vi "HandleObservationSync.vi"(8 "error in (no error)":errorcluster, 11 "S4GUI in":refnum<class "S4GUI.lvclass">) -> (0 "error out":errorcluster, 3 "S4GUI out":refnum<class "S4GUI.lvclass">)   [LabVIEW 2018, in "S4GUI.lvclass"] (continued)
          n1824 = call-dynamic "Read enabled.vi"("error in (no error)"=w5050, "Server in"=w5052) -> ("error out"=w5049:errorcluster, "enabled"=w5048:bool, "Server out"=w5051:refnum<class "Acquisition.lvclass">)  [unwired: 7 in]
          n1825 = case shown="True" w5048 {
            tunnel: [w5106 w5114] -> w5073
            tunnel: [w5107 w5113] -> w5071
            tunnel: w5051 -> [w5107 w5111]
            tunnel: w5049 -> [w5106 w5110]
            frame False {
            }
            frame True {
              n1826 = call-dynamic "Read Channel.vi"("error in (no error)"=w5110, "Acquisition in"=w5111) -> ("error out"=w5118:errorcluster, "Channel.lvclass"=w5119:refnum<class "Channel.lvclass">, "Acquisition out"=w5112:refnum<class "Acquisition.lvclass">)  [unwired: 7 in]
              n1827 = call-dynamic "Read State Machine.vi"("error in (no error)"=w5118, "Device in"=w5119) -> ("error out"=w5117:errorcluster, "State Machine.lvclass"=w5115:refnum<class "State Machine.lvclass">, "Device out"=w5121:refnum<class "Channel.lvclass">)  [unwired: 7 in]
              n1828 = call "Next State.vi"("error in (no error)"=w5117, "New_State"=58, "State Machine in"=w5115) -> ("error out"=w5109:errorcluster, "State Machine out"=w5108:refnum<class "State Machine.lvclass">)  [unwired: 7 in]
              n1829 = call-dynamic "Write State Machine.vi"("error in (no error)"=w5109, "State Machine.lvclass"=w5108, "Device in"=w5121) -> ("error out"=w5122:errorcluster, "Device out"=w5120:refnum<class "Channel.lvclass">)  [unwired: 7 in]
              n1830 = call-dynamic "Write Channel.vi"("error in (no error)"=w5122, "Channel.lvclass"=w5120, "Acquisition in"=w5112) -> ("error out"=w5114:errorcluster, "Acquisition out"=w5113:refnum<class "Acquisition.lvclass">)  [unwired: 7 in]
            }
          }
          n1831 = call-dynamic "Write AcquisitionC.vi"("error in (no error)"=w5073, "Acquisition.lvclass"=w5071, "S4ACS_GUI in"=w5072) -> ("error out"=w5067:errorcluster, "S4ACS_GUI out"=w5066:refnum<class "S4GUI.lvclass">)  [unwired: 7 in]
          n1832 = call-dynamic "Read AcquisitionD.vi"("error in (no error)"=w5067, "S4ACS_GUI in"=w5066) -> ("error out"=w5045:errorcluster, "Acquisition.lvclass"=w5047:refnum<class "Acquisition.lvclass">, "S4ACS_GUI out"=w5065:refnum<class "S4GUI.lvclass">)  [unwired: 7 in]
          n1833 = call-dynamic "Read enabled.vi"("error in (no error)"=w5045, "Server in"=w5047) -> ("error out"=w5044:errorcluster, "enabled"=w5043:bool, "Server out"=w5046:refnum<class "Acquisition.lvclass">)  [unwired: 7 in]
          n1834 = case shown="True" w5043 {
            tunnel: w5044 -> [w5089 w5105]
            tunnel: [w5089 w5104] -> w5068
            tunnel: w5046 -> [w5090 w5095]
            tunnel: [w5090 w5093] -> w5064
            frame False {
            }
            frame True {
              n1835 = call-dynamic "Read Channel.vi"("error in (no error)"=w5105, "Acquisition in"=w5095) -> ("error out"=w5100:errorcluster, "Channel.lvclass"=w5099:refnum<class "Channel.lvclass">, "Acquisition out"=w5094:refnum<class "Acquisition.lvclass">)  [unwired: 7 in]
              n1836 = call-dynamic "Read State Machine.vi"("error in (no error)"=w5100, "Device in"=w5099) -> ("error out"=w5101:errorcluster, "State Machine.lvclass"=w5103:refnum<class "State Machine.lvclass">, "Device out"=w5097:refnum<class "Channel.lvclass">)  [unwired: 7 in]
              n1837 = call "Next State.vi"("error in (no error)"=w5101, "New_State"=58, "State Machine in"=w5103) -> ("error out"=w5091:errorcluster, "State Machine out"=w5092:refnum<class "State Machine.lvclass">)  [unwired: 7 in]
              n1838 = call-dynamic "Write State Machine.vi"("error in (no error)"=w5091, "State Machine.lvclass"=w5092, "Device in"=w5097) -> ("error out"=w5096:errorcluster, "Device out"=w5098:refnum<class "Channel.lvclass">)  [unwired: 7 in]
              n1839 = call-dynamic "Write Channel.vi"("error in (no error)"=w5096, "Channel.lvclass"=w5098, "Acquisition in"=w5094) -> ("error out"=w5104:errorcluster, "Acquisition out"=w5093:refnum<class "Acquisition.lvclass">)  [unwired: 7 in]
            }
          }
          n1840 = call-dynamic "Write AcquisitionD.vi"("error in (no error)"=w5068, "Acquisition.lvclass"=w5064, "S4ACS_GUI in"=w5065) -> ("error out"=w5042:errorcluster, "S4ACS_GUI out"=w5063:refnum<class "S4GUI.lvclass">)  [unwired: 7 in]
          n1841 = flat-sequence {
            tunnel: w5042 -> [w5087]
            tunnel: [w5087] -> w5041
            frame #0 {
              n1842 = Tick Count (ms)() -> (millisecond timer value=→"time9":u32)
            }
          }
          n1843 = Increment(x=w5081) -> (x+1=w5080:u32)
          n1844 = Bundle By Name(cluster=w5063, "Obs_state"=w5080) -> (w5079:refnum<class "S4GUI.lvclass">)
        }
        frame 363 {
          # "T: mode EXPOSE\nF: mode FIRE\nNa seq de foco, só \ndeve usar mode EXPOSE."
          # "Espera todos os canais chegarem ao estado de repouso.\n(estado 0  de Channel:Run.vi)."
          n1845 = call-dynamic "Read AcquisitionA.vi"("error in (no error)"=w5207, "S4ACS_GUI in"=w5208) -> ("error out"=w5186:errorcluster, "Acquisition.lvclass"=w5187:refnum<class "Acquisition.lvclass">, "S4ACS_GUI out"=w5210:refnum<class "S4GUI.lvclass">)  [unwired: 7 in]
          n1846 = call-dynamic "Read enabled.vi"("error in (no error)"=w5186, "Server in"=w5187) -> ("error out"=w5188:errorcluster, "enabled"=w5190:bool, "Server out"=w5189:refnum<class "Acquisition.lvclass">)  [unwired: 7 in]
          n1847 = case shown="True" w5190 {
            tunnel: [w5284 w5302] -> w5211
            tunnel: [w5283 w5301] -> w5209
            tunnel: w5189 -> [w5284 w5294]
            tunnel: w5188 -> [w5283 w5293]
            tunnel: [TRUE w5286] -> w5167
            tunnel: [FALSE w5287] -> w5163
            frame False {
            }
            frame True {
              n1848 = call-dynamic "Read Channel.vi"("error in (no error)"=w5293, "Acquisition in"=w5294) -> ("error out"=w5290:errorcluster, "Channel.lvclass"=w5291:refnum<class "Channel.lvclass">, "Acquisition out"=w5303:refnum<class "Acquisition.lvclass">)  [unwired: 7 in]
              n1849 = call-dynamic "Read wait_expose.vi"("error in (no error)"=w5290, "Channel in"=w5291) -> ("error out"=w5288:errorcluster, "wait_expose"=w5287:bool, "Channel out"=w5289:refnum<class "Channel.lvclass">)  [unwired: 7 in]
              n1850 = call-dynamic "Read State Machine.vi"("error in (no error)"=w5288, "Device in"=w5289) -> ("error out"=w5295:errorcluster, "State Machine.lvclass"=w5297:refnum<class "State Machine.lvclass">, "Device out"=w5299:refnum<class "Channel.lvclass">)  [unwired: 7 in]
              n1851 = call-dynamic "Read State.vi"("error in (no error)"=w5295, "State Machine in"=w5297) -> ("error out"=w5292:errorcluster, "State"=w5285:i32, "State Machine out"=w5296:refnum<class "State Machine.lvclass">)  [unwired: 7 in]
              n1852 = Equal To 0?(x=w5285) -> (x = 0?=w5286:bool)
              n1853 = call-dynamic "Write State Machine.vi"("error in (no error)"=w5292, "State Machine.lvclass"=w5296, "Device in"=w5299) -> ("error out"=w5298:errorcluster, "Device out"=w5300:refnum<class "Channel.lvclass">)  [unwired: 7 in]
              n1854 = call-dynamic "Write Channel.vi"("error in (no error)"=w5298, "Channel.lvclass"=w5300, "Acquisition in"=w5303) -> ("error out"=w5301:errorcluster, "Acquisition out"=w5302:refnum<class "Acquisition.lvclass">)  [unwired: 7 in]
            }
          }
          n1855 = call-dynamic "Write AcquisitionA.vi"("error in (no error)"=w5209, "Acquisition.lvclass"=w5211, "S4ACS_GUI in"=w5210) -> ("error out"=w5203:errorcluster, "S4ACS_GUI out"=w5204:refnum<class "S4GUI.lvclass">)  [unwired: 7 in]
          n1856 = call "Read AcquisitionB.vi"("error in (no error)"=w5203, "S4ACS_GUI in"=w5204) -> ("error out"=w5183:errorcluster, "Acquisition.lvclass"=w5185:refnum<class "Acquisition.lvclass">, "S4ACS_GUI out"=w5201:refnum<class "S4GUI.lvclass">)  [unwired: 7 in]
          n1857 = call-dynamic "Read enabled.vi"("error in (no error)"=w5183, "Server in"=w5185) -> ("error out"=w5182:errorcluster, "enabled"=w5181:bool, "Server out"=w5184:refnum<class "Acquisition.lvclass">)  [unwired: 7 in]
          n1858 = case shown="True" w5181 {
            tunnel: w5184 -> [w5261 w5280]
            tunnel: w5182 -> [w5260 w5279]
            tunnel: [w5261 w5277] -> w5202
            tunnel: [w5260 w5276] -> w5200
            tunnel: [TRUE w5268] -> w5166
            tunnel: [FALSE ("expose") w5262] -> w5162
            frame False {
            }
            frame True {
              n1859 = call-dynamic "Read Channel.vi"("error in (no error)"=w5279, "Acquisition in"=w5280) -> ("error out"=w5264:errorcluster, "Channel.lvclass"=w5266:refnum<class "Channel.lvclass">, "Acquisition out"=w5278:refnum<class "Acquisition.lvclass">)  [unwired: 7 in]
              n1860 = call-dynamic "Read wait_expose.vi"("error in (no error)"=w5264, "Channel in"=w5266) -> ("error out"=w5263:errorcluster, "wait_expose"=w5262:bool, "Channel out"=w5265:refnum<class "Channel.lvclass">)  [unwired: 7 in]
              n1861 = call-dynamic "Read State Machine.vi"("error in (no error)"=w5263, "Device in"=w5265) -> ("error out"=w5270:errorcluster, "State Machine.lvclass"=w5272:refnum<class "State Machine.lvclass">, "Device out"=w5274:refnum<class "Channel.lvclass">)  [unwired: 7 in]
              n1862 = call-dynamic "Read State.vi"("error in (no error)"=w5270, "State Machine in"=w5272) -> ("error out"=w5269:errorcluster, "State"=w5267:i32, "State Machine out"=w5271:refnum<class "State Machine.lvclass">)  [unwired: 7 in]
              n1863 = Equal To 0?(x=w5267) -> (x = 0?=w5268:bool)
              n1864 = call-dynamic "Write State Machine.vi"("error in (no error)"=w5269, "State Machine.lvclass"=w5271, "Device in"=w5274) -> ("error out"=w5273:errorcluster, "Device out"=w5275:refnum<class "Channel.lvclass">)  [unwired: 7 in]
              n1865 = call-dynamic "Write Channel.vi"("error in (no error)"=w5273, "Channel.lvclass"=w5275, "Acquisition in"=w5278) -> ("error out"=w5276:errorcluster, "Acquisition out"=w5277:refnum<class "Acquisition.lvclass">)  [unwired: 7 in]
            }
          }
          n1866 = call "Write AcquisitionB.vi"("error in (no error)"=w5200, "Acquisition.lvclass"=w5202, "S4ACS_GUI in"=w5201) -> ("error out"=w5196:errorcluster, "S4ACS_GUI out"=w5195:refnum<class "S4GUI.lvclass">)  [unwired: 7 in]
          n1867 = call-dynamic "Read AcquisitionC.vi"("error in (no error)"=w5196, "S4ACS_GUI in"=w5195) -> ("error out"=w5178:errorcluster, "Acquisition.lvclass"=w5180:refnum<class "Acquisition.lvclass">, "S4ACS_GUI out"=w5198:refnum<class "S4GUI.lvclass">)  [unwired: 7 in]
          n1868 = call-dynamic "Read enabled.vi"("error in (no error)"=w5178, "Server in"=w5180) -> ("error out"=w5177:errorcluster, "enabled"=w5176:bool, "Server out"=w5179:refnum<class "Acquisition.lvclass">)  [unwired: 7 in]
          n1869 = case shown="True" w5176 {
            tunnel: [w5237 w5252] -> w5199
            tunnel: [w5238 w5251] -> w5197
            tunnel: w5179 -> [w5238 w5247]
            tunnel: w5177 -> [w5237 w5246]
            tunnel: [TRUE w5244] -> w5165
            tunnel: [FALSE ("expose") w5239] -> w5161
            frame False {
            }
            frame True {
              n1870 = call-dynamic "Read Channel.vi"("error in (no error)"=w5246, "Acquisition in"=w5247) -> ("error out"=w5241:errorcluster, "Channel.lvclass"=w5243:refnum<class "Channel.lvclass">, "Acquisition out"=w5250:refnum<class "Acquisition.lvclass">)  [unwired: 7 in]
              n1871 = call-dynamic "Read wait_expose.vi"("error in (no error)"=w5241, "Channel in"=w5243) -> ("error out"=w5240:errorcluster, "wait_expose"=w5239:bool, "Channel out"=w5242:refnum<class "Channel.lvclass">)  [unwired: 7 in]
              n1872 = call-dynamic "Read State Machine.vi"("error in (no error)"=w5240, "Device in"=w5242) -> ("error out"=w5248:errorcluster, "State Machine.lvclass"=w5256:refnum<class "State Machine.lvclass">, "Device out"=w5254:refnum<class "Channel.lvclass">)  [unwired: 7 in]
              n1873 = call-dynamic "Read State.vi"("error in (no error)"=w5248, "State Machine in"=w5256) -> ("error out"=w5249:errorcluster, "State"=w5245:i32, "State Machine out"=w5257:refnum<class "State Machine.lvclass">)  [unwired: 7 in]
              n1874 = Equal To 0?(x=w5245) -> (x = 0?=w5244:bool)
              n1875 = call-dynamic "Write State Machine.vi"("error in (no error)"=w5249, "State Machine.lvclass"=w5257, "Device in"=w5254) -> ("error out"=w5255:errorcluster, "Device out"=w5253:refnum<class "Channel.lvclass">)  [unwired: 7 in]
              n1876 = call-dynamic "Write Channel.vi"("error in (no error)"=w5255, "Channel.lvclass"=w5253, "Acquisition in"=w5250) -> ("error out"=w5252:errorcluster, "Acquisition out"=w5251:refnum<class "Acquisition.lvclass">)  [unwired: 7 in]
            }
          }
          n1877 = call-dynamic "Write AcquisitionC.vi"("error in (no error)"=w5199, "Acquisition.lvclass"=w5197, "S4ACS_GUI in"=w5198) -> ("error out"=w5175:errorcluster, "S4ACS_GUI out"=w5191:refnum<class "S4GUI.lvclass">)  [unwired: 7 in]
          n1878 = call-dynamic "Read AcquisitionD.vi"("error in (no error)"=w5175, "S4ACS_GUI in"=w5191) -> ("error out"=w5171:errorcluster, "Acquisition.lvclass"=w5174:refnum<class "Acquisition.lvclass">, "S4ACS_GUI out"=w5193:refnum<class "S4GUI.lvclass">)  [unwired: 7 in]
          n1879 = call-dynamic "Read enabled.vi"("error in (no error)"=w5171, "Server in"=w5174) -> ("error out"=w5172:errorcluster, "enabled"=w5170:bool, "Server out"=w5173:refnum<class "Acquisition.lvclass">)  [unwired: 7 in]
          n1880 = case shown="True" w5170 {
            tunnel: [w5215 w5233] -> w5194
            tunnel: [w5214 w5232] -> w5192
            tunnel: [TRUE w5222] -> w5164
            tunnel: w5173 -> [w5215 w5224]
            tunnel: w5172 -> [w5214 w5223]
            tunnel: [FALSE ("expose") w5216] -> w5160
            frame False {
            }
            frame True {
              n1881 = call-dynamic "Read Channel.vi"("error in (no error)"=w5223, "Acquisition in"=w5224) -> ("error out"=w5218:errorcluster, "Channel.lvclass"=w5220:refnum<class "Channel.lvclass">, "Acquisition out"=w5234:refnum<class "Acquisition.lvclass">)  [unwired: 7 in]
              n1882 = call-dynamic "Read wait_expose.vi"("error in (no error)"=w5218, "Channel in"=w5220) -> ("error out"=w5217:errorcluster, "wait_expose"=w5216:bool, "Channel out"=w5219:refnum<class "Channel.lvclass">)  [unwired: 7 in]
              n1883 = call-dynamic "Read State Machine.vi"("error in (no error)"=w5217, "Device in"=w5219) -> ("error out"=w5226:errorcluster, "State Machine.lvclass"=w5228:refnum<class "State Machine.lvclass">, "Device out"=w5230:refnum<class "Channel.lvclass">)  [unwired: 7 in]
              n1884 = call-dynamic "Read State.vi"("error in (no error)"=w5226, "State Machine in"=w5228) -> ("error out"=w5225:errorcluster, "State"=w5221:i32, "State Machine out"=w5227:refnum<class "State Machine.lvclass">)  [unwired: 7 in]
              n1885 = Equal To 0?(x=w5221) -> (x = 0?=w5222:bool)
              n1886 = call-dynamic "Write State Machine.vi"("error in (no error)"=w5225, "State Machine.lvclass"=w5227, "Device in"=w5230) -> ("error out"=w5229:errorcluster, "Device out"=w5231:refnum<class "Channel.lvclass">)  [unwired: 7 in]
              n1887 = call-dynamic "Write Channel.vi"("error in (no error)"=w5229, "Channel.lvclass"=w5231, "Acquisition in"=w5234) -> ("error out"=w5232:errorcluster, "Acquisition out"=w5233:refnum<class "Acquisition.lvclass">)  [unwired: 7 in]
            }
          }
          n1888 = call-dynamic "Write AcquisitionD.vi"("error in (no error)"=w5192, "Acquisition.lvclass"=w5194, "S4ACS_GUI in"=w5193) -> ("error out"=w5158:errorcluster, "S4ACS_GUI out"=w5159:refnum<class "S4GUI.lvclass">)  [unwired: 7 in]
          n1889 = Compound Arithmetic op=OR(w5163, w5162, w5161, w5160) -> ()  [unwired: 1 out]
          n1890 = Compound Arithmetic op=AND(w5167, w5166, w5165, w5164) -> (w5168:bool)
          n1891 = Increment(x=w5169) -> (x+1=w5157:u32)
          n1892 = Select(t=w5157, s=w5168, f=w5169) -> (s? t:f=w5205:u32)
          n1893 = Bundle By Name(cluster=w5159, "Obs_state"=w5205) -> (w5206:refnum<class "S4GUI.lvclass">)
        }
        frame 364 {
          n1894 = flat-sequence {
            tunnel: [w5317] -> w5305
            tunnel: w5306 -> [w5317]
            tunnel: [w5313] -> w5304
            frame #0 {
              # "Espera 2s desde que enviou o comando\nWRITE_HEADER_DATA para os ACS"
              n1895 = local read "time9"() -> (w5312:u32)
              n1896 = Tick Count (ms)() -> (millisecond timer value=w5316:u32)
              "time 10" <- w5316
              n1897 = Subtract(x=w5316, y=w5312) -> (x-y=w5315:u32)
              "delay 89" <- w5315
              n1898 = Greater?(x=w5315, y=u32 2000) -> (0:w5313:bool)
            }
          }
          n1899 = Increment(x=w5309) -> (x+1=w5308:u32)
          n1900 = Select(t=w5308, s=w5304, f=w5309) -> (s? t:f=w5310:u32)
          n1901 = Bundle By Name(cluster=w5307, "Obs_state"=w5310) -> (w5311:refnum<class "S4GUI.lvclass">)
        }
        frame 365 {
          n1902 = call-dynamic "Read AcquisitionA.vi"("error in (no error)"=w5358, "S4ACS_GUI in"=w5359) -> ("error out"=w5334:errorcluster, "Acquisition.lvclass"=w5337:refnum<class "Acquisition.lvclass">, "S4ACS_GUI out"=w5361:refnum<class "S4GUI.lvclass">)  [unwired: 7 in]
          n1903 = call-dynamic "Read enabled.vi"("error in (no error)"=w5334, "Server in"=w5337) -> ("error out"=w5333:errorcluster, "enabled"=w5335:bool, "Server out"=w5336:refnum<class "Acquisition.lvclass">)  [unwired: 7 in]
          n1904 = case shown="True" w5335 {
            tunnel: w5336 -> [w5415 w5430]
            tunnel: w5333 -> [w5414 w5429]
            tunnel: [w5415 w5427] -> w5362
            tunnel: [w5414 w5426] -> w5360
            frame False {
            }
            frame True {
              n1905 = call-dynamic "Read Channel.vi"("error in (no error)"=w5429, "Acquisition in"=w5430) -> ("error out"=w5422:errorcluster, "Channel.lvclass"=w5421:refnum<class "Channel.lvclass">, "Acquisition out"=w5428:refnum<class "Acquisition.lvclass">)  [unwired: 7 in]
              n1906 = call-dynamic "Read State Machine.vi"("error in (no error)"=w5422, "Device in"=w5421) -> ("error out"=w5423:errorcluster, "State Machine.lvclass"=w5425:refnum<class "State Machine.lvclass">, "Device out"=w5419:refnum<class "Channel.lvclass">)  [unwired: 7 in]
              n1907 = call "Next State.vi"("error in (no error)"=w5423, "New_State"=50, "State Machine in"=w5425) -> ("error out"=w5416:errorcluster, "State Machine out"=w5417:refnum<class "State Machine.lvclass">)  [unwired: 7 in]
              n1908 = call-dynamic "Write State Machine.vi"("error in (no error)"=w5416, "State Machine.lvclass"=w5417, "Device in"=w5419) -> ("error out"=w5418:errorcluster, "Device out"=w5420:refnum<class "Channel.lvclass">)  [unwired: 7 in]
              n1909 = call-dynamic "Write Channel.vi"("error in (no error)"=w5418, "Channel.lvclass"=w5420, "Acquisition in"=w5428) -> ("error out"=w5426:errorcluster, "Acquisition out"=w5427:refnum<class "Acquisition.lvclass">)  [unwired: 7 in]
            }
          }
          n1910 = call-dynamic "Write AcquisitionA.vi"("error in (no error)"=w5360, "Acquisition.lvclass"=w5362, "S4ACS_GUI in"=w5361) -> ("error out"=w5353:errorcluster, "S4ACS_GUI out"=w5354:refnum<class "S4GUI.lvclass">)  [unwired: 7 in]
          n1911 = call "Read AcquisitionB.vi"("error in (no error)"=w5353, "S4ACS_GUI in"=w5354) -> ("error out"=w5330:errorcluster, "Acquisition.lvclass"=w5332:refnum<class "Acquisition.lvclass">, "S4ACS_GUI out"=w5351:refnum<class "S4GUI.lvclass">)  [unwired: 7 in]
          n1912 = call-dynamic "Read enabled.vi"("error in (no error)"=w5330, "Server in"=w5332) -> ("error out"=w5329:errorcluster, "enabled"=w5328:bool, "Server out"=w5331:refnum<class "Acquisition.lvclass">)  [unwired: 7 in]
          n1913 = case shown="True" w5328 {
            tunnel: w5331 -> [w5398 w5413]
            tunnel: w5329 -> [w5397 w5412]
            tunnel: [w5398 w5410] -> w5352
            tunnel: [w5397 w5409] -> w5350
            frame False {
            }
            frame True {
              n1914 = call-dynamic "Read Channel.vi"("error in (no error)"=w5412, "Acquisition in"=w5413) -> ("error out"=w5405:errorcluster, "Channel.lvclass"=w5404:refnum<class "Channel.lvclass">, "Acquisition out"=w5411:refnum<class "Acquisition.lvclass">)  [unwired: 7 in]
              n1915 = call-dynamic "Read State Machine.vi"("error in (no error)"=w5405, "Device in"=w5404) -> ("error out"=w5406:errorcluster, "State Machine.lvclass"=w5408:refnum<class "State Machine.lvclass">, "Device out"=w5402:refnum<class "Channel.lvclass">)  [unwired: 7 in]
              n1916 = call "Next State.vi"("error in (no error)"=w5406, "New_State"=50, "State Machine in"=w5408) -> ("error out"=w5399:errorcluster, "State Machine out"=w5400:refnum<class "State Machine.lvclass">)  [unwired: 7 in]
              n1917 = call-dynamic "Write State Machine.vi"("error in (no error)"=w5399, "State Machine.lvclass"=w5400, "Device in"=w5402) -> ("error out"=w5401:errorcluster, "Device out"=w5403:refnum<class "Channel.lvclass">)  [unwired: 7 in]
              n1918 = call-dynamic "Write Channel.vi"("error in (no error)"=w5401, "Channel.lvclass"=w5403, "Acquisition in"=w5411) -> ("error out"=w5409:errorcluster, "Acquisition out"=w5410:refnum<class "Acquisition.lvclass">)  [unwired: 7 in]
            }
          }
          n1919 = call "Write AcquisitionB.vi"("error in (no error)"=w5350, "Acquisition.lvclass"=w5352, "S4ACS_GUI in"=w5351) -> ("error out"=w5346:errorcluster, "S4ACS_GUI out"=w5345:refnum<class "S4GUI.lvclass">)  [unwired: 7 in]
          n1920 = call-dynamic "Read AcquisitionC.vi"("error in (no error)"=w5346, "S4ACS_GUI in"=w5345) -> ("error out"=w5325:errorcluster, "Acquisition.lvclass"=w5327:refnum<class "Acquisition.lvclass">, "S4ACS_GUI out"=w5348:refnum<class "S4GUI.lvclass">)  [unwired: 7 in]
          n1921 = call-dynamic "Read enabled.vi"("error in (no error)"=w5325, "Server in"=w5327) -> ("error out"=w5324:errorcluster, "enabled"=w5323:bool, "Server out"=w5326:refnum<class "Acquisition.lvclass">)  [unwired: 7 in]
          n1922 = case shown="True" w5323 {
            tunnel: [w5380 w5388] -> w5349
            tunnel: [w5381 w5387] -> w5347
            tunnel: w5326 -> [w5381 w5385]
            tunnel: w5324 -> [w5380 w5384]
            frame False {
            }
            frame True {
              n1923 = call-dynamic "Read Channel.vi"("error in (no error)"=w5384, "Acquisition in"=w5385) -> ("error out"=w5392:errorcluster, "Channel.lvclass"=w5393:refnum<class "Channel.lvclass">, "Acquisition out"=w5386:refnum<class "Acquisition.lvclass">)  [unwired: 7 in]
              n1924 = call-dynamic "Read State Machine.vi"("error in (no error)"=w5392, "Device in"=w5393) -> ("error out"=w5391:errorcluster, "State Machine.lvclass"=w5389:refnum<class "State Machine.lvclass">, "Device out"=w5395:refnum<class "Channel.lvclass">)  [unwired: 7 in]
              n1925 = call "Next State.vi"("error in (no error)"=w5391, "New_State"=50, "State Machine in"=w5389) -> ("error out"=w5383:errorcluster, "State Machine out"=w5382:refnum<class "State Machine.lvclass">)  [unwired: 7 in]
              n1926 = call-dynamic "Write State Machine.vi"("error in (no error)"=w5383, "State Machine.lvclass"=w5382, "Device in"=w5395) -> ("error out"=w5396:errorcluster, "Device out"=w5394:refnum<class "Channel.lvclass">)  [unwired: 7 in]
              n1927 = call-dynamic "Write Channel.vi"("error in (no error)"=w5396, "Channel.lvclass"=w5394, "Acquisition in"=w5386) -> ("error out"=w5388:errorcluster, "Acquisition out"=w5387:refnum<class "Acquisition.lvclass">)  [unwired: 7 in]
            }
          }
          n1928 = call-dynamic "Write AcquisitionC.vi"("error in (no error)"=w5349, "Acquisition.lvclass"=w5347, "S4ACS_GUI in"=w5348) -> ("error out"=w5343:errorcluster, "S4ACS_GUI out"=w5342:refnum<class "S4GUI.lvclass">)  [unwired: 7 in]
          n1929 = call-dynamic "Read AcquisitionD.vi"("error in (no error)"=w5343, "S4ACS_GUI in"=w5342) -> ("error out"=w5320:errorcluster, "Acquisition.lvclass"=w5322:refnum<class "Acquisition.lvclass">, "S4ACS_GUI out"=w5341:refnum<class "S4GUI.lvclass">)  [unwired: 7 in]
          n1930 = call-dynamic "Read enabled.vi"("error in (no error)"=w5320, "Server in"=w5322) -> ("error out"=w5319:errorcluster, "enabled"=w5318:bool, "Server out"=w5321:refnum<class "Acquisition.lvclass">)  [unwired: 7 in]
          n1931 = case shown="True" w5318 {
            tunnel: w5319 -> [w5363 w5379]
            tunnel: [w5363 w5378] -> w5344
            tunnel: w5321 -> [w5364 w5369]
            tunnel: [w5364 w5367] -> w5340
            frame False {
            }
            frame True {
              n1932 = call-dynamic "Read Channel.vi"("error in (no error)"=w5379, "Acquisition in"=w5369) -> ("error out"=w5374:errorcluster, "Channel.lvclass"=w5373:refnum<class "Channel.lvclass">, "Acquisition out"=w5368:refnum<class "Acquisition.lvclass">)  [unwired: 7 in]
              n1933 = call-dynamic "Read State Machine.vi"("error in (no error)"=w5374, "Device in"=w5373) -> ("error out"=w5375:errorcluster, "State Machine.lvclass"=w5377:refnum<class "State Machine.lvclass">, "Device out"=w5371:refnum<class "Channel.lvclass">)  [unwired: 7 in]
              n1934 = call "Next State.vi"("error in (no error)"=w5375, "New_State"=50, "State Machine in"=w5377) -> ("error out"=w5365:errorcluster, "State Machine out"=w5366:refnum<class "State Machine.lvclass">)  [unwired: 7 in]
              n1935 = call-dynamic "Write State Machine.vi"("error in (no error)"=w5365, "State Machine.lvclass"=w5366, "Device in"=w5371) -> ("error out"=w5370:errorcluster, "Device out"=w5372:refnum<class "Channel.lvclass">)  [unwired: 7 in]
              n1936 = call-dynamic "Write Channel.vi"("error in (no error)"=w5370, "Channel.lvclass"=w5372, "Acquisition in"=w5368) -> ("error out"=w5378:errorcluster, "Acquisition out"=w5367:refnum<class "Acquisition.lvclass">)  [unwired: 7 in]
            }
          }
          n1937 = call-dynamic "Write AcquisitionD.vi"("error in (no error)"=w5344, "Acquisition.lvclass"=w5340, "S4ACS_GUI in"=w5341) -> ("error out"=w5339:errorcluster, "S4ACS_GUI out"=w5338:refnum<class "S4GUI.lvclass">)  [unwired: 7 in]
          n1938 = Increment(x=w5357) -> (x+1=w5356:u32)
          n1939 = Bundle By Name(cluster=w5338, "Obs_state"=w5356) -> (w5355:refnum<class "S4GUI.lvclass">)
        }
        frame 366 {
          # "Espera todos os canais com CyclesDone=0"
          # "Espera todos os canais chegarem ao estado ACTIVE\n(estados 54 e 55 de Channel:Run.vi)."
          n1940 = call-dynamic "Read AcquisitionA.vi"("error in (no error)"=w5482, "S4ACS_GUI in"=w5483) -> ("error out"=w5461:errorcluster, "Acquisition.lvclass"=w5462:refnum<class "Acquisition.lvclass">, "S4ACS_GUI out"=w5485:refnum<class "S4GUI.lvclass">)  [unwired: 7 in]
          n1941 = call-dynamic "Read enabled.vi"("error in (no error)"=w5461, "Server in"=w5462) -> ("error out"=w5463:errorcluster, "enabled"=w5465:bool, "Server out"=w5464:refnum<class "Acquisition.lvclass">)  [unwired: 7 in]
          n1942 = case shown="True" w5465 {
            tunnel: [w5562 w5581] -> w5486
            tunnel: [w5561 w5580] -> w5484
            tunnel: w5464 -> [w5562 w5573]
            tunnel: w5463 -> [w5561 w5572]
            tunnel: [TRUE w5571] -> w5443
            tunnel: [u32 0 ("CyclesDone") w5563] -> w5435
            frame False {
            }
            frame True {
              n1943 = call-dynamic "Read Channel.vi"("error in (no error)"=w5572, "Acquisition in"=w5573) -> ("error out"=w5566:errorcluster, "Channel.lvclass"=w5567:refnum<class "Channel.lvclass">, "Acquisition out"=w5582:refnum<class "Acquisition.lvclass">)  [unwired: 7 in]
              n1944 = call-dynamic "Read CyclesDone.vi"("error in (no error)"=w5566, "Channel in"=w5567) -> ("error out"=w5564:errorcluster, "CyclesDone"=w5563:u32, "Channel out"=w5565:refnum<class "Channel.lvclass">)  [unwired: 7 in]
              n1945 = call-dynamic "Read State Machine.vi"("error in (no error)"=w5564, "Device in"=w5565) -> ("error out"=w5574:errorcluster, "State Machine.lvclass"=w5576:refnum<class "State Machine.lvclass">, "Device out"=w5578:refnum<class "Channel.lvclass">)  [unwired: 7 in]
              n1946 = call-dynamic "Read State.vi"("error in (no error)"=w5574, "State Machine in"=w5576) -> ("error out"=w5568:errorcluster, "State"=w5570:i32, "State Machine out"=w5575:refnum<class "State Machine.lvclass">)  [unwired: 7 in]
              n1947 = Greater?(x=w5570, y=53) -> (0:w5571:bool)
              n1948 = call-dynamic "Write State Machine.vi"("error in (no error)"=w5568, "State Machine.lvclass"=w5575, "Device in"=w5578) -> ("error out"=w5577:errorcluster, "Device out"=w5579:refnum<class "Channel.lvclass">)  [unwired: 7 in]
              n1949 = call-dynamic "Write Channel.vi"("error in (no error)"=w5577, "Channel.lvclass"=w5579, "Acquisition in"=w5582) -> ("error out"=w5580:errorcluster, "Acquisition out"=w5581:refnum<class "Acquisition.lvclass">)  [unwired: 7 in]
            }
          }
          n1950 = call-dynamic "Write AcquisitionA.vi"("error in (no error)"=w5484, "Acquisition.lvclass"=w5486, "S4ACS_GUI in"=w5485) -> ("error out"=w5478:errorcluster, "S4ACS_GUI out"=w5479:refnum<class "S4GUI.lvclass">)  [unwired: 7 in]
          n1951 = call "Read AcquisitionB.vi"("error in (no error)"=w5478, "S4ACS_GUI in"=w5479) -> ("error out"=w5458:errorcluster, "Acquisition.lvclass"=w5460:refnum<class "Acquisition.lvclass">, "S4ACS_GUI out"=w5476:refnum<class "S4GUI.lvclass">)  [unwired: 7 in]
          n1952 = call-dynamic "Read enabled.vi"("error in (no error)"=w5458, "Server in"=w5460) -> ("error out"=w5457:errorcluster, "enabled"=w5456:bool, "Server out"=w5459:refnum<class "Acquisition.lvclass">)  [unwired: 7 in]
          n1953 = case shown="True" w5456 {
            tunnel: w5459 -> [w5538 w5558]
            tunnel: w5457 -> [w5537 w5557]
            tunnel: [w5538 w5555] -> w5477
            tunnel: [w5537 w5554] -> w5475
            tunnel: [TRUE w5545] -> w5442
            tunnel: [u32 0 ("CyclesDone") w5539] -> w5436
            frame False {
            }
            frame True {
              n1954 = call-dynamic "Read Channel.vi"("error in (no error)"=w5557, "Acquisition in"=w5558) -> ("error out"=w5541:errorcluster, "Channel.lvclass"=w5543:refnum<class "Channel.lvclass">, "Acquisition out"=w5556:refnum<class "Acquisition.lvclass">)  [unwired: 7 in]
              n1955 = call-dynamic "Read CyclesDone.vi"("error in (no error)"=w5541, "Channel in"=w5543) -> ("error out"=w5540:errorcluster, "CyclesDone"=w5539:u32, "Channel out"=w5542:refnum<class "Channel.lvclass">)  [unwired: 7 in]
              n1956 = call-dynamic "Read State Machine.vi"("error in (no error)"=w5540, "Device in"=w5542) -> ("error out"=w5548:errorcluster, "State Machine.lvclass"=w5550:refnum<class "State Machine.lvclass">, "Device out"=w5552:refnum<class "Channel.lvclass">)  [unwired: 7 in]
              n1957 = call-dynamic "Read State.vi"("error in (no error)"=w5548, "State Machine in"=w5550) -> ("error out"=w5547:errorcluster, "State"=w5544:i32, "State Machine out"=w5549:refnum<class "State Machine.lvclass">)  [unwired: 7 in]
              n1958 = Greater?(x=w5544, y=53) -> (0:w5545:bool)
              n1959 = call-dynamic "Write State Machine.vi"("error in (no error)"=w5547, "State Machine.lvclass"=w5549, "Device in"=w5552) -> ("error out"=w5551:errorcluster, "Device out"=w5553:refnum<class "Channel.lvclass">)  [unwired: 7 in]
              n1960 = call-dynamic "Write Channel.vi"("error in (no error)"=w5551, "Channel.lvclass"=w5553, "Acquisition in"=w5556) -> ("error out"=w5554:errorcluster, "Acquisition out"=w5555:refnum<class "Acquisition.lvclass">)  [unwired: 7 in]
            }
          }
          n1961 = call "Write AcquisitionB.vi"("error in (no error)"=w5475, "Acquisition.lvclass"=w5477, "S4ACS_GUI in"=w5476) -> ("error out"=w5471:errorcluster, "S4ACS_GUI out"=w5470:refnum<class "S4GUI.lvclass">)  [unwired: 7 in]
          n1962 = call-dynamic "Read AcquisitionC.vi"("error in (no error)"=w5471, "S4ACS_GUI in"=w5470) -> ("error out"=w5453:errorcluster, "Acquisition.lvclass"=w5455:refnum<class "Acquisition.lvclass">, "S4ACS_GUI out"=w5473:refnum<class "S4GUI.lvclass">)  [unwired: 7 in]
          n1963 = call-dynamic "Read enabled.vi"("error in (no error)"=w5453, "Server in"=w5455) -> ("error out"=w5452:errorcluster, "enabled"=w5451:bool, "Server out"=w5454:refnum<class "Acquisition.lvclass">)  [unwired: 7 in]
          n1964 = case shown="True" w5451 {
            tunnel: [w5513 w5529] -> w5474
            tunnel: [w5514 w5528] -> w5472
            tunnel: w5454 -> [w5514 w5524]
            tunnel: w5452 -> [w5513 w5523]
            tunnel: [TRUE w5520] -> w5441
            tunnel: [u32 0 ("CyclesDone") w5515] -> w5434
            frame False {
            }
            frame True {
              n1965 = call-dynamic "Read Channel.vi"("error in (no error)"=w5523, "Acquisition in"=w5524) -> ("error out"=w5517:errorcluster, "Channel.lvclass"=w5519:refnum<class "Channel.lvclass">, "Acquisition out"=w5527:refnum<class "Acquisition.lvclass">)  [unwired: 7 in]
              n1966 = call-dynamic "Read CyclesDone.vi"("error in (no error)"=w5517, "Channel in"=w5519) -> ("error out"=w5516:errorcluster, "CyclesDone"=w5515:u32, "Channel out"=w5518:refnum<class "Channel.lvclass">)  [unwired: 7 in]
              n1967 = call-dynamic "Read State Machine.vi"("error in (no error)"=w5516, "Device in"=w5518) -> ("error out"=w5525:errorcluster, "State Machine.lvclass"=w5533:refnum<class "State Machine.lvclass">, "Device out"=w5531:refnum<class "Channel.lvclass">)  [unwired: 7 in]
              n1968 = call-dynamic "Read State.vi"("error in (no error)"=w5525, "State Machine in"=w5533) -> ("error out"=w5526:errorcluster, "State"=w5521:i32, "State Machine out"=w5534:refnum<class "State Machine.lvclass">)  [unwired: 7 in]
              n1969 = Greater?(x=w5521, y=53) -> (0:w5520:bool)
              n1970 = call-dynamic "Write State Machine.vi"("error in (no error)"=w5526, "State Machine.lvclass"=w5534, "Device in"=w5531) -> ("error out"=w5532:errorcluster, "Device out"=w5530:refnum<class "Channel.lvclass">)  [unwired: 7 in]
              n1971 = call-dynamic "Write Channel.vi"("error in (no error)"=w5532, "Channel.lvclass"=w5530, "Acquisition in"=w5527) -> ("error out"=w5529:errorcluster, "Acquisition out"=w5528:refnum<class "Acquisition.lvclass">)  [unwired: 7 in]
            }
          }
          n1972 = call-dynamic "Write AcquisitionC.vi"("error in (no error)"=w5474, "Acquisition.lvclass"=w5472, "S4ACS_GUI in"=w5473) -> ("error out"=w5450:errorcluster, "S4ACS_GUI out"=w5466:refnum<class "S4GUI.lvclass">)  [unwired: 7 in]
          n1973 = call-dynamic "Read AcquisitionD.vi"("error in (no error)"=w5450, "S4ACS_GUI in"=w5466) -> ("error out"=w5446:errorcluster, "Acquisition.lvclass"=w5449:refnum<class "Acquisition.lvclass">, "S4ACS_GUI out"=w5468:refnum<class "S4GUI.lvclass">)  [unwired: 7 in]
          n1974 = call-dynamic "Read enabled.vi"("error in (no error)"=w5446, "Server in"=w5449) -> ("error out"=w5447:errorcluster, "enabled"=w5445:bool, "Server out"=w5448:refnum<class "Acquisition.lvclass">)  [unwired: 7 in]
          n1975 = case shown="True" w5445 {
            tunnel: [w5490 w5509] -> w5469
            tunnel: [w5489 w5508] -> w5467
            tunnel: [TRUE w5497] -> w5440
            tunnel: w5448 -> [w5490 w5500]
            tunnel: w5447 -> [w5489 w5499]
            tunnel: [u32 0 ("CyclesDone") w5491] -> w5433
            frame False {
            }
            frame True {
              n1976 = call-dynamic "Read Channel.vi"("error in (no error)"=w5499, "Acquisition in"=w5500) -> ("error out"=w5493:errorcluster, "Channel.lvclass"=w5495:refnum<class "Channel.lvclass">, "Acquisition out"=w5510:refnum<class "Acquisition.lvclass">)  [unwired: 7 in]
              n1977 = call-dynamic "Read CyclesDone.vi"("error in (no error)"=w5493, "Channel in"=w5495) -> ("error out"=w5492:errorcluster, "CyclesDone"=w5491:u32, "Channel out"=w5494:refnum<class "Channel.lvclass">)  [unwired: 7 in]
              n1978 = call-dynamic "Read State Machine.vi"("error in (no error)"=w5492, "Device in"=w5494) -> ("error out"=w5502:errorcluster, "State Machine.lvclass"=w5504:refnum<class "State Machine.lvclass">, "Device out"=w5506:refnum<class "Channel.lvclass">)  [unwired: 7 in]
              n1979 = call-dynamic "Read State.vi"("error in (no error)"=w5502, "State Machine in"=w5504) -> ("error out"=w5501:errorcluster, "State"=w5496:i32, "State Machine out"=w5503:refnum<class "State Machine.lvclass">)  [unwired: 7 in]
              n1980 = Greater?(x=w5496, y=53) -> (0:w5497:bool)
              n1981 = call-dynamic "Write State Machine.vi"("error in (no error)"=w5501, "State Machine.lvclass"=w5503, "Device in"=w5506) -> ("error out"=w5505:errorcluster, "Device out"=w5507:refnum<class "Channel.lvclass">)  [unwired: 7 in]
              n1982 = call-dynamic "Write Channel.vi"("error in (no error)"=w5505, "Channel.lvclass"=w5507, "Acquisition in"=w5510) -> ("error out"=w5508:errorcluster, "Acquisition out"=w5509:refnum<class "Acquisition.lvclass">)  [unwired: 7 in]
            }
          }
          n1983 = call-dynamic "Write AcquisitionD.vi"("error in (no error)"=w5467, "Acquisition.lvclass"=w5469, "S4ACS_GUI in"=w5468) -> ("error out"=w5438:errorcluster, "S4ACS_GUI out"=w5439:refnum<class "S4GUI.lvclass">)  [unwired: 7 in]
          n1984 = Compound Arithmetic op=AND(w5443, w5442, w5441, w5440) -> ()  [unwired: 1 out]
          n1985 = Compound Arithmetic op=ADD(w5435, w5436, w5434, w5433) -> (w5432:u32)
          n1986 = Equal To 0?(x=w5432) -> (x = 0?=w5431:bool)
          n1987 = Increment(x=w5444) -> (x+1=w5437:u32)
          n1988 = Select(t=w5437, s=w5431, f=w5444) -> (s? t:f=w5480:u32)
          n1989 = Bundle By Name(cluster=w5439, "Obs_state"=w5480) -> (w5481:refnum<class "S4GUI.lvclass">)
        }
        frame 367 {
          # "T=canais receberam STOP"
          # "OV 2024.01.26 DEBUG - ignora os ciclos!!\nT= Todos os canais ativos no mesmo ciclo;\nF= Canais com ciclo diferente"
          # "T= Todos os canais ativos na mesma sequencia;\nF= Canais com sequencia diferente"
          # "Todos os CYCLES_DONE \nmudaram e são iguais?\nSe sim, avança a lâmina."
          n1990 = Unbundle By Name(w5618) -> ("cyclesDone"=w5612:u32)
          n1991 = call-dynamic "Read AcquisitionA.vi"("error in (no error)"=w5653, "S4ACS_GUI in"=w5618) -> ("error out"=w5633:errorcluster, "Acquisition.lvclass"=w5634:refnum<class "Acquisition.lvclass">, "S4ACS_GUI out"=w5655:refnum<class "S4GUI.lvclass">)  [unwired: 7 in]
          n1992 = call-dynamic "Read enabled.vi"("error in (no error)"=w5633, "Server in"=w5634) -> ("error out"=w5632:errorcluster, "enabled"=w5600:bool, "Server out"=w5631:refnum<class "Acquisition.lvclass">)  [unwired: 7 in]
          n1993 = case shown="True" w5600 {
            tunnel: w5632 -> [w5870 w5889]
            tunnel: [w5871 w5887] -> w5656
            tunnel: [w5870 w5886] -> w5654
            tunnel: [u32 0 ("SequesDone") w5885] -> w5606
            tunnel: w5631 -> [w5871 w5884]
            tunnel: w5612 -> [_ w5883]
            tunnel: [TRUE w5882] -> w5617
            tunnel: [u32 0 ("CubesDone") w5881] -> w5593
            tunnel: [FALSE ("stopping") w5872] -> w5589
            frame False {
            }
            frame True {
              # "CYCLES_DONE = 0->1"
              n1994 = call-dynamic "Read Channel.vi"("error in (no error)"=w5889, "Acquisition in"=w5884) -> ("error out"=w5878:errorcluster, "Channel.lvclass"=w5880:refnum<class "Channel.lvclass">, "Acquisition out"=w5888:refnum<class "Acquisition.lvclass">)  [unwired: 7 in]
              n1995 = call-dynamic "Read CyclesDone.vi"("error in (no error)"=w5878, "Channel in"=w5880) -> ("error out"=w5877:errorcluster, "CyclesDone"=w5881:u32, "Channel out"=w5879:refnum<class "Channel.lvclass">)  [unwired: 7 in]
              n1996 = call-dynamic "Read CyclesDone.vi"("error in (no error)"=w5877, "Channel in"=w5879) -> ("error out"=w5875:errorcluster, "CyclesDone"=w5885:u32, "Channel out"=w5876:refnum<class "Channel.lvclass">)  [unwired: 7 in]
              n1997 = Not Equal?(x=w5885, y=w5883) -> (x != y?=w5882:bool)
              n1998 = call-dynamic "Read stopping.vi"("error in (no error)"=w5875, "Channel in"=w5876) -> ("error out"=w5874:errorcluster, "stopping"=w5872:bool, "Channel out"=w5873:refnum<class "Channel.lvclass">)  [unwired: 7 in]
              n1999 = call-dynamic "Write Channel.vi"("error in (no error)"=w5874, "Channel.lvclass"=w5873, "Acquisition in"=w5888) -> ("error out"=w5886:errorcluster, "Acquisition out"=w5887:refnum<class "Acquisition.lvclass">)  [unwired: 7 in]
            }
          }
          n2000 = call-dynamic "Write AcquisitionA.vi"("error in (no error)"=w5654, "Acquisition.lvclass"=w5656, "S4ACS_GUI in"=w5655) -> ("error out"=w5650:errorcluster, "S4ACS_GUI out"=w5649:refnum<class "S4GUI.lvclass">)  [unwired: 7 in]
          n2001 = call "Read AcquisitionB.vi"("error in (no error)"=w5650, "S4ACS_GUI in"=w5649) -> ("error out"=w5627:errorcluster, "Acquisition.lvclass"=w5630:refnum<class "Acquisition.lvclass">, "S4ACS_GUI out"=w5651:refnum<class "S4GUI.lvclass">)  [unwired: 7 in]
          n2002 = call-dynamic "Read enabled.vi"("error in (no error)"=w5627, "Server in"=w5630) -> ("error out"=w5628:errorcluster, "enabled"=w5599:bool, "Server out"=w5629:refnum<class "Acquisition.lvclass">)  [unwired: 7 in]
          n2003 = case shown="True" w5599 {
            tunnel: w5628 -> [w5846 w5865]
            tunnel: w5629 -> [w5847 w5864]
            tunnel: [u32 0 ("SequesDone") w5859] -> w5603
            tunnel: [w5846 w5863] -> w5648
            tunnel: [w5847 w5862] -> w5647
            tunnel: w5612 -> [_ w5858]
            tunnel: [TRUE w5857] -> w5613
            tunnel: [u32 0 ("CubesDone") w5852] -> w5592
            tunnel: [FALSE ("stopping") w5848] -> w5588
            frame False {
            }
            frame True {
              n2004 = call-dynamic "Read Channel.vi"("error in (no error)"=w5865, "Acquisition in"=w5864) -> ("error out"=w5854:errorcluster, "Channel.lvclass"=w5856:refnum<class "Channel.lvclass">, "Acquisition out"=w5860:refnum<class "Acquisition.lvclass">)  [unwired: 7 in]
              n2005 = call-dynamic "Read CyclesDone.vi"("error in (no error)"=w5854, "Channel in"=w5856) -> ("error out"=w5853:errorcluster, "CyclesDone"=w5852:u32, "Channel out"=w5855:refnum<class "Channel.lvclass">)  [unwired: 7 in]
              n2006 = call-dynamic "Read CyclesDone.vi"("error in (no error)"=w5853, "Channel in"=w5855) -> ("error out"=w5850:errorcluster, "CyclesDone"=w5859:u32, "Channel out"=w5861:refnum<class "Channel.lvclass">)  [unwired: 7 in]
              n2007 = Not Equal?(x=w5859, y=w5858) -> (x != y?=w5857:bool)
              n2008 = call-dynamic "Read stopping.vi"("error in (no error)"=w5850, "Channel in"=w5861) -> ("error out"=w5849:errorcluster, "stopping"=w5848:bool, "Channel out"=w5851:refnum<class "Channel.lvclass">)  [unwired: 7 in]
              n2009 = call-dynamic "Write Channel.vi"("error in (no error)"=w5849, "Channel.lvclass"=w5851, "Acquisition in"=w5860) -> ("error out"=w5863:errorcluster, "Acquisition out"=w5862:refnum<class "Acquisition.lvclass">)  [unwired: 7 in]
            }
          }
          n2010 = Max & Min(x=w5593, y=w5592) -> (max(x,y)=w5609:u32)  [unwired: 1 out]
          n2011 = Max & Min(x=w5606, y=w5603) -> (max(x,y)=w5616:u32)  [unwired: 1 out]
          n2012 = call "Write AcquisitionB.vi"("error in (no error)"=w5648, "Acquisition.lvclass"=w5647, "S4ACS_GUI in"=w5651) -> ("error out"=w5640:errorcluster, "S4ACS_GUI out"=w5639:refnum<class "S4GUI.lvclass">)  [unwired: 7 in]
          n2013 = call-dynamic "Read AcquisitionC.vi"("error in (no error)"=w5640, "S4ACS_GUI in"=w5639) -> ("error out"=w5624:errorcluster, "Acquisition.lvclass"=w5626:refnum<class "Acquisition.lvclass">, "S4ACS_GUI out"=w5642:refnum<class "S4GUI.lvclass">)  [unwired: 7 in]
          n2014 = call-dynamic "Read enabled.vi"("error in (no error)"=w5624, "Server in"=w5626) -> ("error out"=w5623:errorcluster, "enabled"=w5598:bool, "Server out"=w5625:refnum<class "Acquisition.lvclass">)  [unwired: 7 in]
          n2015 = case shown="True" w5598 {
            tunnel: [w5822 w5841] -> w5643
            tunnel: [w5823 w5840] -> w5641
            tunnel: w5623 -> [w5822 w5837]
            tunnel: w5625 -> [w5823 w5838]
            tunnel: [u32 0 ("SequesDone") w5836] -> w5602
            tunnel: w5612 -> [_ w5835]
            tunnel: [TRUE w5834] -> w5611
            tunnel: [u32 0 ("CubesDone") w5828] -> w5591
            tunnel: [FALSE ("stopping") w5824] -> w5587
            frame False {
            }
            frame True {
              n2016 = call-dynamic "Read Channel.vi"("error in (no error)"=w5837, "Acquisition in"=w5838) -> ("error out"=w5830:errorcluster, "Channel.lvclass"=w5832:refnum<class "Channel.lvclass">, "Acquisition out"=w5839:refnum<class "Acquisition.lvclass">)  [unwired: 7 in]
              n2017 = call-dynamic "Read CyclesDone.vi"("error in (no error)"=w5830, "Channel in"=w5832) -> ("error out"=w5829:errorcluster, "CyclesDone"=w5828:u32, "Channel out"=w5831:refnum<class "Channel.lvclass">)  [unwired: 7 in]
              n2018 = call-dynamic "Read CyclesDone.vi"("error in (no error)"=w5829, "Channel in"=w5831) -> ("error out"=w5826:errorcluster, "CyclesDone"=w5836:u32, "Channel out"=w5833:refnum<class "Channel.lvclass">)  [unwired: 7 in]
              n2019 = Not Equal?(x=w5836, y=w5835) -> (x != y?=w5834:bool)
              n2020 = call-dynamic "Read stopping.vi"("error in (no error)"=w5826, "Channel in"=w5833) -> ("error out"=w5825:errorcluster, "stopping"=w5824:bool, "Channel out"=w5827:refnum<class "Channel.lvclass">)  [unwired: 7 in]
              n2021 = call-dynamic "Write Channel.vi"("error in (no error)"=w5825, "Channel.lvclass"=w5827, "Acquisition in"=w5839) -> ("error out"=w5841:errorcluster, "Acquisition out"=w5840:refnum<class "Acquisition.lvclass">)  [unwired: 7 in]
            }
          }
          n2022 = call-dynamic "Write AcquisitionC.vi"("error in (no error)"=w5643, "Acquisition.lvclass"=w5641, "S4ACS_GUI in"=w5642) -> ("error out"=w5637:errorcluster, "S4ACS_GUI out"=w5638:refnum<class "S4GUI.lvclass">)  [unwired: 7 in]
          n2023 = call-dynamic "Read AcquisitionD.vi"("error in (no error)"=w5637, "S4ACS_GUI in"=w5638) -> ("error out"=w5620:errorcluster, "Acquisition.lvclass"=w5622:refnum<class "Acquisition.lvclass">, "S4ACS_GUI out"=w5644:refnum<class "S4GUI.lvclass">)  [unwired: 7 in]
          n2024 = call-dynamic "Read enabled.vi"("error in (no error)"=w5620, "Server in"=w5622) -> ("error out"=w5619:errorcluster, "enabled"=w5597:bool, "Server out"=w5621:refnum<class "Acquisition.lvclass">)  [unwired: 7 in]
          n2025 = Build Array(w5600, w5599, w5598, w5597) -> (w5596:bool[])
          n2026 = case shown="True" w5597 {
            tunnel: [w5799 w5817] -> w5646
            tunnel: [w5798 w5816] -> w5645
            tunnel: w5621 -> [w5799 w5815]
            tunnel: w5619 -> [w5798 w5814]
            tunnel: [u32 0 ("SequesDone") w5812] -> w5605
            tunnel: w5612 -> [_ w5811]
            tunnel: [TRUE w5810] -> w5610
            tunnel: [u32 0 ("CubesDone") w5804] -> w5590
            tunnel: [FALSE ("stopping") w5800] -> w5586
            frame False {
            }
            frame True {
              n2027 = call-dynamic "Read Channel.vi"("error in (no error)"=w5814, "Acquisition in"=w5815) -> ("error out"=w5806:errorcluster, "Channel.lvclass"=w5808:refnum<class "Channel.lvclass">, "Acquisition out"=w5813:refnum<class "Acquisition.lvclass">)  [unwired: 7 in]
              n2028 = call-dynamic "Read CyclesDone.vi"("error in (no error)"=w5806, "Channel in"=w5808) -> ("error out"=w5805:errorcluster, "CyclesDone"=w5804:u32, "Channel out"=w5807:refnum<class "Channel.lvclass">)  [unwired: 7 in]
              n2029 = call-dynamic "Read CyclesDone.vi"("error in (no error)"=w5805, "Channel in"=w5807) -> ("error out"=w5802:errorcluster, "CyclesDone"=w5812:u32, "Channel out"=w5809:refnum<class "Channel.lvclass">)  [unwired: 7 in]
              n2030 = Not Equal?(x=w5812, y=w5811) -> (x != y?=w5810:bool)
              n2031 = call-dynamic "Read stopping.vi"("error in (no error)"=w5802, "Channel in"=w5809) -> ("error out"=w5801:errorcluster, "stopping"=w5800:bool, "Channel out"=w5803:refnum<class "Channel.lvclass">)  [unwired: 7 in]
              n2032 = call-dynamic "Write Channel.vi"("error in (no error)"=w5801, "Channel.lvclass"=w5803, "Acquisition in"=w5813) -> ("error out"=w5816:errorcluster, "Acquisition out"=w5817:refnum<class "Acquisition.lvclass">)  [unwired: 7 in]
            }
          }
          n2033 = Boolean Array To Number(Boolean array=w5596) -> (number=w5594:u32)
          n2034 = Max & Min(x=w5591, y=w5590) -> (max(x,y)=w5608:u32)  [unwired: 1 out]
          n2035 = Max & Min(x=w5602, y=w5605) -> (max(x,y)=w5615:u32)  [unwired: 1 out]
          n2036 = Compound Arithmetic op=AND(w5617, w5613, w5611, w5610) -> (w5595:bool)
          n2037 = Max & Min(x=w5616, y=w5615) -> (max(x,y)=w5614:u32)  [unwired: 1 out]
          n2038 = Max & Min(x=w5609, y=w5608) -> (max(x,y)=w5607:u32)  [unwired: 1 out]
          n2039 = case shown="12" w5594 {
            tunnel: w5593 -> [w5664 _ w5676 _ w5685 _ w5691 w5697 _ w5703 w5706 _]
            tunnel: w5590 -> [w5663 w5667 w5672 w5679 w5680 w5688 w5690 _ _ _ _ _]
            tunnel: w5592 -> [w5662 w5665 _ _ w5684 w5686 _ w5696 w5700 _ w5705 _]
            tunnel: w5591 -> [w5661 w5666 w5671 w5677 _ _ _ w5695 w5699 w5702 _ _]
            tunnel: [w5657 w5668 w5673 w5678 w5681 w5687 w5689 w5692 w5698 w5701 w5704 TRUE] -> _
            frame 15 {
              # "A,B,C,D ativos"
              n2040 = Equal?(x=w5664, y=w5662) -> (x = y?=w5660:bool)
              n2041 = Equal?(x=w5661, y=w5663) -> (x = y?=w5658:bool)
              n2042 = Equal?(x=w5662, y=w5661) -> (x = y?=w5659:bool)
              n2043 = Compound Arithmetic op=AND(w5660, w5659, w5658) -> (w5657:bool)
            }
            frame 14 {
              # "B,C e,D ativos"
              n2044 = Equal?(x=w5665, y=w5666) -> (x = y?=w5670:bool)
              n2045 = Equal?(x=w5666, y=w5667) -> (x = y?=w5669:bool)
              n2046 = Compound Arithmetic op=AND(w5670, w5669) -> (w5668:bool)
            }
            frame 13 {
              # "A,C e,D ativos"
              n2047 = Equal?(x=w5676, y=w5671) -> (x = y?=w5675:bool)
              n2048 = Equal?(x=w5671, y=w5672) -> (x = y?=w5674:bool)
              n2049 = Compound Arithmetic op=AND(w5675, w5674) -> (w5673:bool)
            }
            frame 12 {
              # "Só C e D ativos"
              n2050 = Equal?(x=w5677, y=w5679) -> (x = y?=w5678:bool)
            }
            frame 11 {
              # "A,B e,D ativos"
              n2051 = Equal?(x=w5685, y=w5684) -> (x = y?=w5683:bool)
              n2052 = Equal?(x=w5684, y=w5680) -> (x = y?=w5682:bool)
              n2053 = Compound Arithmetic op=AND(w5683, w5682) -> (w5681:bool)
            }
            frame 10 {
              # "Só B e D ativos"
              n2054 = Equal?(x=w5686, y=w5688) -> (x = y?=w5687:bool)
            }
            frame 9 {
              # "Só A e D ativos"
              n2055 = Equal?(x=w5691, y=w5690) -> (x = y?=w5689:bool)
            }
            frame 7 {
              # "A,B,C ativos"
              n2056 = Equal?(x=w5697, y=w5696) -> (x = y?=w5694:bool)
              n2057 = Equal?(x=w5696, y=w5695) -> (x = y?=w5693:bool)
              n2058 = Compound Arithmetic op=AND(w5694, w5693) -> (w5692:bool)
            }
            frame 6 {
              # "Só B e C ativos"
              n2059 = Equal?(x=w5700, y=w5699) -> (x = y?=w5698:bool)
            }
            frame 5 {
              # "Só A e C ativos"
              n2060 = Equal?(x=w5703, y=w5702) -> (x = y?=w5701:bool)
            }
            frame 3 {
              # "só A e B ativos"
              n2061 = Equal?(x=w5706, y=w5705) -> (x = y?=w5704:bool)
            }
            frame 0..2, 4, 8, Default {
              # "nenhum ou só 1  \ncanal ativo."
            }
          }
          n2062 = Compound Arithmetic op=OR(w5589, w5588, w5587, w5586) -> (w5585:bool)
          n2063 = case shown="0..2, 4, 8, Default" w5594 {
            tunnel: w5606 -> [w5715 _ w5727 _ w5736 _ w5742 w5748 _ w5754 w5757 _]
            tunnel: w5605 -> [w5714 w5718 w5723 w5730 w5731 w5739 w5741 _ _ _ _ _]
            tunnel: w5603 -> [w5713 w5716 _ _ w5735 w5737 _ w5747 w5751 _ w5756 _]
            tunnel: w5602 -> [w5712 w5717 w5722 w5728 _ _ _ w5746 w5750 w5753 _ _]
            tunnel: [w5708 w5719 w5724 w5729 w5732 w5738 w5740 w5743 w5749 w5752 w5755 TRUE] -> w5601
            frame 15 {
              # "A,B,C,D ativos"
              n2064 = Equal?(x=w5715, y=w5713) -> (x = y?=w5711:bool)
              n2065 = Equal?(x=w5712, y=w5714) -> (x = y?=w5709:bool)
              n2066 = Equal?(x=w5713, y=w5712) -> (x = y?=w5710:bool)
              n2067 = Compound Arithmetic op=AND(w5711, w5710, w5709) -> (w5708:bool)
            }
            frame 14 {
              # "B,C e,D ativos"
              n2068 = Equal?(x=w5716, y=w5717) -> (x = y?=w5721:bool)
              n2069 = Equal?(x=w5717, y=w5718) -> (x = y?=w5720:bool)
              n2070 = Compound Arithmetic op=AND(w5721, w5720) -> (w5719:bool)
            }
            frame 13 {
              # "A,C e,D ativos"
              n2071 = Equal?(x=w5727, y=w5722) -> (x = y?=w5726:bool)
              n2072 = Equal?(x=w5722, y=w5723) -> (x = y?=w5725:bool)
              n2073 = Compound Arithmetic op=AND(w5726, w5725) -> (w5724:bool)
            }
            frame 12 {
              # "Só C e D ativos"
              n2074 = Equal?(x=w5728, y=w5730) -> (x = y?=w5729:bool)
            }
            frame 11 {
              # "A,B e,D ativos"
              n2075 = Equal?(x=w5736, y=w5735) -> (x = y?=w5734:bool)
              n2076 = Equal?(x=w5735, y=w5731) -> (x = y?=w5733:bool)
              n2077 = Compound Arithmetic op=AND(w5734, w5733) -> (w5732:bool)
            }
            frame 10 {
              # "Só B e D ativos"
              n2078 = Equal?(x=w5737, y=w5739) -> (x = y?=w5738:bool)
            }
            frame 9 {
              # "Só A e D ativos"
              n2079 = Equal?(x=w5742, y=w5741) -> (x = y?=w5740:bool)
            }
            frame 7 {
              # "A,B,C ativos"
              n2080 = Equal?(x=w5748, y=w5747) -> (x = y?=w5745:bool)
              n2081 = Equal?(x=w5747, y=w5746) -> (x = y?=w5744:bool)
              n2082 = Compound Arithmetic op=AND(w5745, w5744) -> (w5743:bool)
            }
            frame 6 {
              # "Só B e C ativos"
              n2083 = Equal?(x=w5751, y=w5750) -> (x = y?=w5749:bool)
            }
            frame 5 {
              # "Só A e C ativos"
              n2084 = Equal?(x=w5754, y=w5753) -> (x = y?=w5752:bool)
            }
            frame 3 {
              # "só A e B ativos"
              n2085 = Equal?(x=w5757, y=w5756) -> (x = y?=w5755:bool)
            }
            frame 0..2, 4, 8, Default {
              # "nenhum ou só 1  \ncanal ativo."
            }
          }
          n2086 = call-dynamic "Write AcquisitionD.vi"("error in (no error)"=w5645, "Acquisition.lvclass"=w5646, "S4ACS_GUI in"=w5644) -> ("error out"=w5635:errorcluster, "S4ACS_GUI out"=w5636:refnum<class "S4GUI.lvclass">)  [unwired: 7 in]
          n2087 = And(x=w5595, y=w5601) -> (x .and. y?=w5604:bool)
          n2088 = case shown="True" w5604 {
            tunnel: w5636 -> [w5760 w5772]
            tunnel: [w5759 w5771] -> w5652
            tunnel: w5614 -> [_ w5770]
            tunnel: w5607 -> [_ _]
            tunnel: w5595 -> [w5761 _]
            tunnel: TRUE -> [_ w5769]
            tunnel: w5585 -> [_ w5768]
            tunnel: w5583 -> [_ w5767]
            frame False {
              n2089 = case shown="True" w5761 {
                tunnel: w5760 -> [w5762 w5766]
                tunnel: [w5762 w5765] -> w5759
                frame False {
                }
                frame True {
                  n2090 = Bundle By Name(cluster=w5766, "Obs_state"=u32 1, "Error Msg"="ERROR: Sequence_done not equal in all active channels.") -> (w5765:refnum<class "S4GUI.lvclass">)
                }
              }
            }
            frame True {
              n2091 = case shown="True" w5769 {
                tunnel: w5772 -> [w5774 w5784]
                tunnel: [w5773 w5783] -> w5771
                tunnel: w5770 -> [_ w5782]
                tunnel: w5768 -> [_ w5778]
                tunnel: w5767 -> [_ w5777]
                frame False {
                  n2092 = Bundle By Name(cluster=w5774, "Obs_state"=u32 1, "Error Msg"="ERROR: Cycles_done not equal in all active channels.") -> (w5773:refnum<class "S4GUI.lvclass">)
                }
                frame True {
                  # "STOP?"
                  n2093 = local read "time308"() -> (w5780:u32)
                  n2094 = Tick Count (ms)() -> (millisecond timer value=w5781:u32)
                  n2095 = Subtract(x=w5781, y=w5780) -> (x-y=→"delay Acq 2":u32)
                  n2096 = case shown="False" w5778 {
                    tunnel: w5784 -> [w5788 w5793]
                    tunnel: [w5787 w5792] -> w5783
                    tunnel: w5782 -> [w5785 w5789]
                    tunnel: w5777 -> [_ w5791]
                    frame True {
                      n2097 = Bundle By Name(cluster=w5788, "Obs_state"=u32 0, "sequesDone"=w5785, "cyclesDone"=w5785) -> (w5787:refnum<class "S4GUI.lvclass">)
                    }
                    frame False {
                      n2098 = Increment(x=w5791) -> (x+1=w5790:u32)
